vi "GV_StartStop.vi"() -> ()   [LabVIEW 2023]
panel:
  out "Numeric":i32
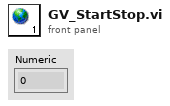
[diagram p1: front panel]
diagram:
